vi "DFD Plot Narrowband Freq Response.vi"(6 "fs [Hz]":dbl=-1.0 format="%.2f", 7 "# freq bins":i32=-1, 8 "error in (no error)":errorcluster, 9 "dB on? (T)":bool=TRUE, 10 "phase view":T7, 11 "narrowband filter in":T1 {"multirate filters"."mMRate_SumWl" min=1 max=32 step=1; "multirate filters"."mMRate_InputIwl" min=1 max=32 step=1; "multirate filters"."mMRate_GainWl" min=1 max=32 step=1; "multirate filters"."mMRate_OutputWl" min=1 max=32 step=1; "multirate filters"."mMRate_InputWl" min=1 max=32 step=1; "multirate filters"."mMRate_CoefWl" min=1 max=32 step=1; "multirate filters"."mMRate_Mode" items=["Default"=-1, "No Rate Change"=0, "Interpolation"=1, "Decimation"=2, "Interpolated"=3, "Rational"=4]}) -> (0 "error out":errorcluster, 1 "phase response":cluster{"f0":dbl, "df":dbl, "phase":dbl[]}(graph), 2 "magnitude response":cluster{"f0":dbl, "df":dbl, "magnitude":dbl[]}(graph), 3 "narrowband filter out":T1 {"multirate filters"."mMRate_SumWl" min=1 max=32 step=1; "multirate filters"."mMRate_InputIwl" min=1 max=32 step=1; "multirate filters"."mMRate_GainWl" min=1 max=32 step=1; "multirate filters"."mMRate_OutputWl" min=1 max=32 step=1; "multirate filters"."mMRate_InputWl" min=1 max=32 step=1; "multirate filters"."mMRate_CoefWl" min=1 max=32 step=1; "multirate filters"."mMRate_Mode" items=["Default"=-1, "No Rate Change"=0, "Interpolation"=1, "Decimation"=2, "Interpolated"=3, "Rational"=4]})   [LabVIEW 2017, in "NI_DigFilterLicensed.lvlib"]
doc: "Plots the frequency responses, including the magnitude and phase responses, of a narrowband filter."
uses:
  <vilib>/addons/Digital Filter Design/NI_DigFilterLicensed.lvlib
  <vilib>/addons/Digital Filter Design/_Objects.llb/DFD Narrowband Filter Obj.ctl
  <vilib>/addons/Digital Filter Design/_Objects.llb/DFD Multirate Filter Obj.ctl
  <vilib>/addons/Digital Filter Design/_Objects.llb/DFD Multirate Mode.ctl
  <vilib>/addons/Digital Filter Design/_Objects.llb/DFD Coef Norm Type.ctl
  <vilib>/addons/Digital Filter Design/_Objects.llb/DFD Round-off Mode.ctl
  <vilib>/addons/Digital Filter Design/_Objects.llb/DFD FXP MRate Multiply Mode.ctl
  <vilib>/addons/Digital Filter Design/_Objects.llb/DFD Phase Setting.ctl
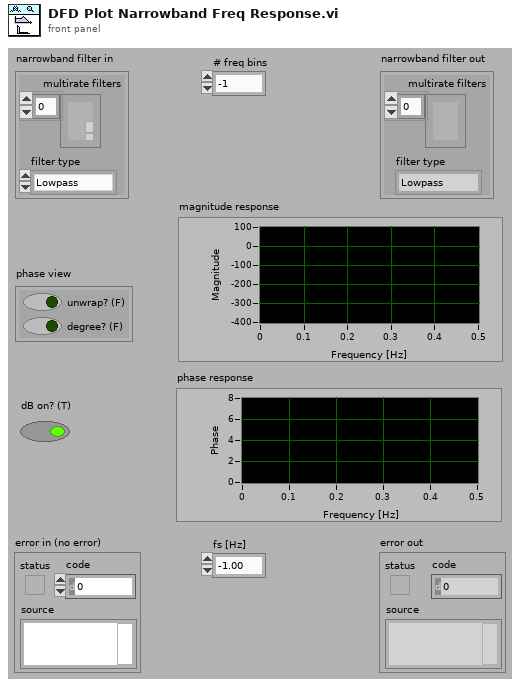
[diagram p1: front panel]
types:
  T1 = typedef "NI_DigFilterLicensed.lvlib/DFD Narrowband Filter Obj.ctl" = cluster{"multirate filters":T2[], "filter type":enum32{"Lowpass", "Highpass", "Bandpass", "Bandstop", "Wideband-Lowpass", "Wideband-Highpass"}}
  T2 = typedef "NI_DigFilterLicensed.lvlib/DFD Multirate Filter Obj.ctl" = cluster{"mMRate_Structure":enum16{"CIC", "FIR", "IIR", "Lattice"}, "mMRate_Mode":T3, "mMRate_Factor":i32, "mMRate_FIRParams":cluster{"mMRate_FIR_H":dbl[], "mMRate_FIR_IsNyquist?":bool, "mMRate_FIR_IsSymmetric?":bool}, "mMRate_CICParams":cluster{"mMRate_CIC_#Stage":i32, "mMRate_CIC_Lag":i32, "mMRate_CIC_Type":enum16{"Lowpass", "Highpass"}}, "mMRate_Order":i32, "mMRate_Version":string, "mMRate_Comments":string, "mMRate_RationalFactor":cluster{"mMRate_L":i32, "mMRate_M":i32}, "mMRate_Fs":dbl, "mMRate_Quantized?":bool, "mMRate_QFilterGain":dbl, "mMRate_CoefWl":i16, "mMRate_Scaling":cluster{"mMRate_ScaleByPowerOf2?":bool, "mMRate_ScaleType":T4}, "mMRate_InputWl":i16, "mMRate_OutputWl":i16, "mMRate_OutputMode":T5, "mMRate_MultMode":T6, "mMRate_BitPruning":bool, "mMRate_GainWl":i16, "mMRate_OutputFwl":i16, "mMRate_SumIwl":i16, "mMRate_InputIwl ":i16, "mMRate_SumWl":i16, "mMRate_CoefIwl":i16}
  T3 = typedef "NI_DigFilterLicensed.lvlib/DFD Multirate Mode.ctl" = i16
  T4 = typedef "NI_DigFilterLicensed.lvlib/DFD Coef Norm Type.ctl" = enum16{"No Norm", "Time Domain 1-Norm", "Time Domain 2-Norm", "Time Domain Inf-Norm"}
  T5 = typedef "NI_DigFilterLicensed.lvlib/DFD Round-off Mode.ctl" = enum16{"Nearest", "Truncation"}
  T6 = typedef "NI_DigFilterLicensed.lvlib/DFD FXP MRate Multiply Mode.ctl" = enum16{"Truncated", "Full"}
  T7 = typedef "NI_DigFilterLicensed.lvlib/DFD Phase Setting.ctl" = cluster{"unwrap? (F)":bool, "degree? (F)":bool}
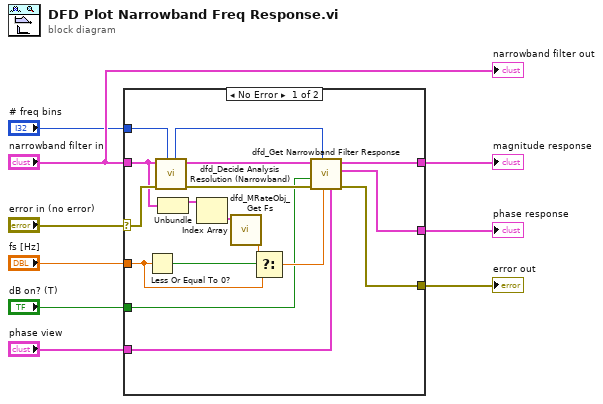
[diagram p0: block diagram]
diagram:
  n1 = case shown="No Error" "error in (no error)" {
    selector: "error in (no error)" -> [w21 w27]
    tunnel: "narrowband filter in" -> [w13 _]
    tunnel: "fs [Hz]" -> [w25 _]
    tunnel: "dB on? (T)" -> [w16 _]
    tunnel: "phase view" -> [w15 _]
    tunnel: [w22 w27] -> w5
    tunnel: [w24 _] -> w3
    tunnel: [w23 _] -> w2
    tunnel: "# freq bins" -> [w19 _]
    frame No Error {
      n2 = Less Or Equal To 0?(x=w25) -> (x <= 0?=w26:bool)
      n3 = call <vilib>:"dfd_Decide Analysis Resolution (Narrowband).vi"("# freq bins in"=w19, "error in (no error)"=w21, "narrowband filter in"=w13) -> ("error out"=w20:errorcluster, "narrowband filter out"=w18:T1, "# freq bins out"=w14:i32)  [unwired: 6 out]
      n4 = Unbundle(w13) -> ("multirate filters"=w12:T2[])  [unwired: 1 out]
      n5 = Index Array(array=w12) -> (element=w11:T2)  [unwired: 1 in]
      n6 = call <vilib>:"dfd_MRateObj_Get Fs.vi"("multirate filter in"=w11) -> ("fs"=w10:dbl)  [unwired: 10 out]
      n7 = Select(t=w10, s=w26, f=w25) -> (s? t:f=w17:dbl)
      n8 = call <vilib>:"dfd_Get Narrowband Filter Response.vi"("phase view"=w15, "fs in [Hz]"=w17, "# freq bins"=w14, "error in (no error)"=w20, "dB on? (T)"=w16, "narrowband filter in"=w18) -> ("error out"=w22:errorcluster, "phase response"=w23:cluster{"f0":dbl, "df":dbl, "phase":dbl[]}, "magnitude response"=w24:cluster{"f0":dbl, "df":dbl, "magnitude":dbl[]})  [unwired: 3 out]
    }
    frame Error {
    }
  }
  "error out" <- w5
  "magnitude response" <- w3
  "phase response" <- w2
  "narrowband filter out" <- "narrowband filter in"
